vi "Rinocloud_image_upload.vi"(5 "Extra metadata array":T1(array[cluster])=[{"Attribute"="", "Value"="", "Data type"=enum."<null>"}], 6 "Notes":string, 7 "Tags":string, 8 "error in (no error)":errorcluster, 9 "Wavefrom Refnum":refnum<vi>, 10 "Name":string, 11 "Parent ID":string) -> (0 "error out":errorcluster, 1 "Saved":bool, 2 "body":string, 3 "headers":string)   [LabVIEW 2011, in "Rinocloud Library.lvlib"]
uses:
  Rinocloud Library.lvlib
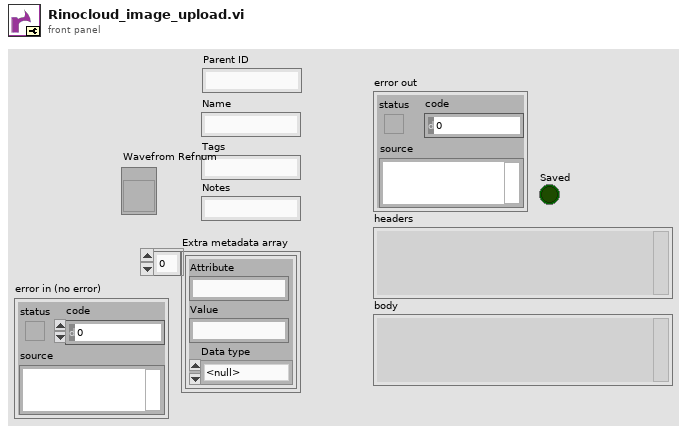
[diagram p1: front panel]
types:
  T1 = cluster{"Attribute":string, "Value":string, "Data type":enum16{"Numeric", "String", "1D array of strings", "1D array of doubles", "Data JSON string", "<null>"}}[]
  T2 = typedef "imagedata.ctl" = cluster{"image type":i32, "image depth":i32, "image":u8[], "mask":u8[], "colors":u32[], "Rectangle":cluster{"left":i16, "top":i16, "right":i16, "bottom":i16}}
  T3 = cluster{"headers":string, "body":string, "ID":string, "Saved":bool}
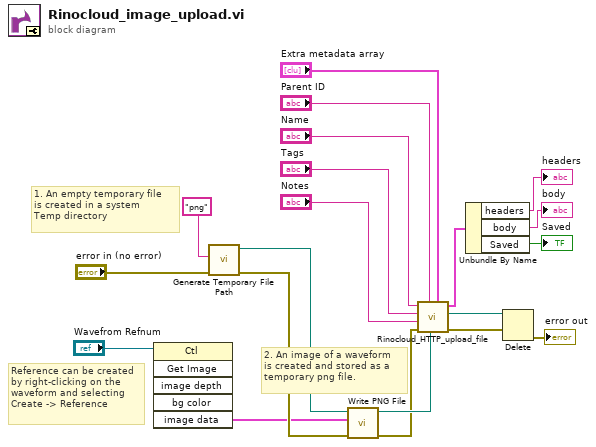
[diagram p0: block diagram]
diagram:
  # "Reference can be created\nby right-clicking on the\nwaveform and selecting \nCreate -> Reference"
  # "2. An image of a waveform\nis created and stored as a\ntemporary png file."
  # "1. An empty temporary file \nis created in a system \nTemp directory"
  n1 = invoke class="Ctl" method="Get Image"(reference="Wavefrom Refnum") -> ("image data"=w15:T2)  [unwired: 5 in, 5 out]
  n2 = call <vilib>:"Generate Temporary File Path.vi"("error in (no error)"="error in (no error)", "Temporary File Extension (tmp)"="png" ("name or relative path")) -> ("error out"=w17:errorcluster, "Unique Temporary File Path"=w18:path)  [unwired: 8 in]
  n3 = call <vilib>:"Write PNG File.vi"("error in (no error)"=w17, "image data"=w15, "path to PNG file"=w18) -> ("error out"=w1:errorcluster, "path"=w6:path)  [unwired: 7 in]
  n4 = call "Rinocloud_HTTP_upload_file.vi"("Extra metadata array"="Extra metadata array", "Path in"=w6, "Parent ID"="Parent ID", "error in (no error)"=w1, "Notes"="Notes", "Tags"="Tags", "Name"="Name") -> ("error out"=w2:errorcluster, "Path out"=w5:path, "Status"=w9:T3)  [unwired: 2 in]
  n5 = Unbundle By Name(w9) -> ("headers"=→"headers":string, "body"=→"body":string, "Saved"=→"Saved":bool)
  n6 = Delete(path (use dialog)=w5, error in=w2) -> (error out=→"error out":errorcluster)  [unwired: 3 in, 2 out]
